vi "Read Arduino String.vi"(8 "error in (no error)":errorcluster, 11 "reference":refnum<visa-resource-name>) -> (0 "error out":errorcluster, 2 "response":string, 3 "reference out":refnum<visa-resource-name>)   [LabVIEW 2021, in "FW Arduino Control.lvclass"]
uses:
  FW Arduino Control.lvclass
  c4a16319-bda1-49ab-9101-4525acf5d1d2.vi
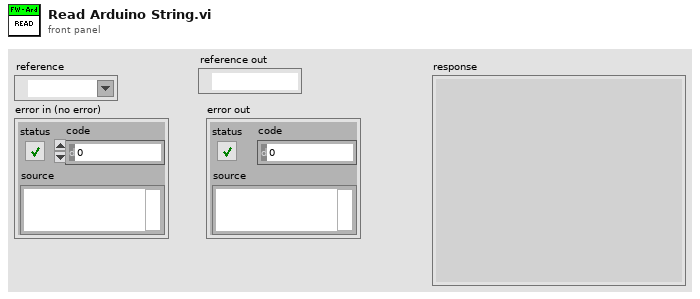
[diagram p1: front panel]
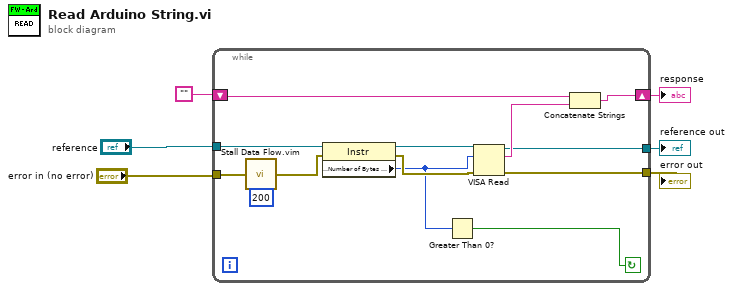
[diagram p0: block diagram]
diagram:
  n1 = while {
    tunnel: "reference" -> [w19]
    tunnel: "error in (no error)" -> [w17]
    shift-right: [w11] -> w3
    shift-left: "" -> [w12]
    tunnel: [w8] -> w2
    tunnel: [w7] -> w1
    stop <- w9 continue-if-true
    n2 = call "Stall Data Flow.vim"("value in"=w17, "milliseconds to wait"=u32 200) -> ("value out"=w16:errorcluster)  [unwired: 1 out]
    n3 = property class="Instr"(reference=w19, error in=w16) -> (reference out=w18:refnum<visa-resource-name>, error out=w14:errorcluster, "Serial Settings:Number of Bytes at Serial Port"=w10:u32)
    n4 = Greater Than 0?(x=w10) -> (x > 0?=w9:bool)
    n5 = VISA Read(VISA resource name=w18, byte count=w10, error in (no error)=w14) -> (VISA resource name out=w8:refnum<visa-resource-name>, read buffer=w13:string, error out=w7:errorcluster)  [unwired: 1 out]
    n6 = Concatenate Strings(w12, w13) -> (w11:string)
  }
  "response" <- w3
  "reference out" <- w2
  "error out" <- w1
